vi "Response_Status.vi"(8 "error in (no error)":errorcluster, 11 "Response in":refnum<class "Response.lvclass">) -> (0 "error out":errorcluster, 1 "Status Description":string, 2 "Status Code":dbl, 3 "Response out":refnum<class "Response.lvclass">)   [LabVIEW 2016, in "Response.lvclass"]
uses:
  Response.lvclass
  Response.lvclass/Response.ctl
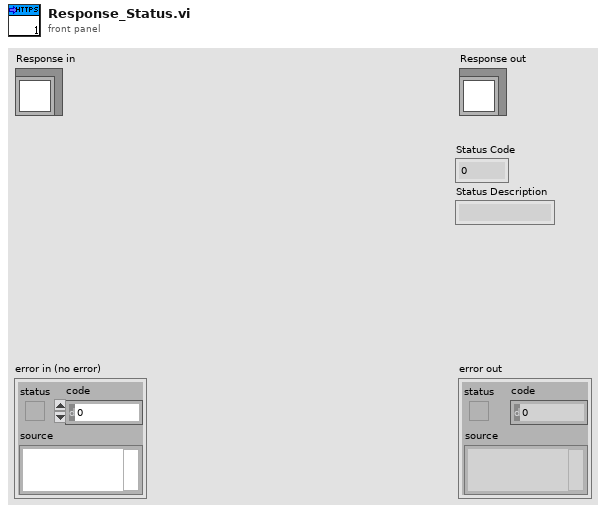
[diagram p1: front panel]
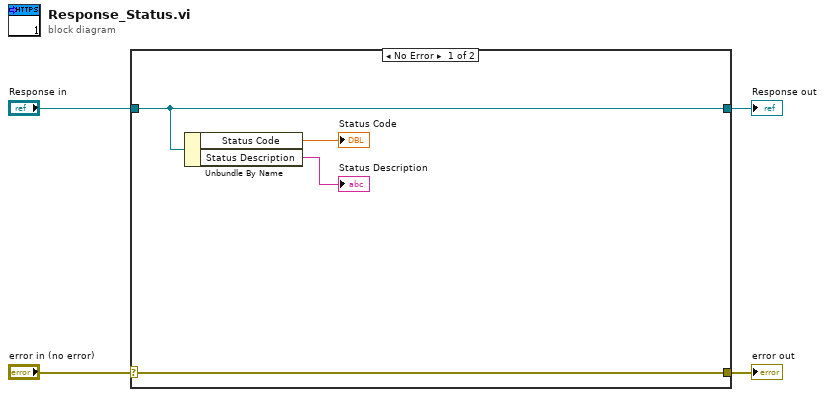
[diagram p0: block diagram]
diagram:
  n1 = case shown="No Error" "error in (no error)" {
    selector: "error in (no error)" -> [w8 w10]
    tunnel: [w8 w10] -> w3
    tunnel: [w7 w9] -> w1
    tunnel: "Response in" -> [w7 w9]
    frame No Error {
      n2 = Unbundle By Name(w7) -> ("Status Code"=→"Status Code":dbl, "Status Description"=→"Status Description":string)
    }
    frame Error {
    }
  }
  "error out" <- w3
  "Response out" <- w1
